vi "F Dwf Digital In Status Samples Left.vi"(8 "error in (no error)":errorcluster, 10 "pcSamplesLeft":i32, 11 "hdwf":i32) -> (0 "error out":errorcluster, 2 "pcSamplesLeft out":i32, 3 "function return":i32)   [LabVIEW 2019, in "Olasdwf.lvlib"]
doc: "DWFAPI int FDwfDigitalInStatusSamplesLeft(HDWF hdwf, int *pcSamplesLeft);"
uses:
  Olasdwf.lvlib
  Windows/System32/dwf.dll
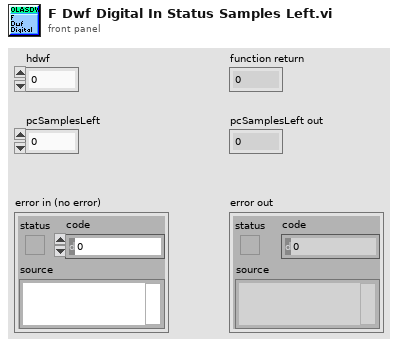
[diagram p1: front panel]
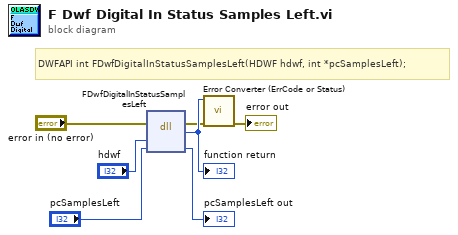
[diagram p0: block diagram]
diagram:
  # "DWFAPI int FDwfDigitalInStatusSamplesLeft(HDWF hdwf, int *pcSamplesLeft);"
  n1 = dll-call lib="C:/Windows/System32/dwf.*" fn="FDwfDigitalInStatusSamplesLeft"(error in="error in (no error)", "hdwf"="hdwf", "pcSamplesLeft"="pcSamplesLeft") -> (error out=w2:errorcluster, w7:i32, "pcSamplesLeft"=→"pcSamplesLeft out":i32)  [unwired: 3 in, 1 out]
  "function return" <- w7
  n2 = call "Error Converter (ErrCode or Status).vi"("error in (no error)"=w2, "error code"=w7) -> ("error out"=→"error out":errorcluster)  [unwired: 9 in]
